vi "Filter Names by Suffix.vi"(8 "Error In":errorcluster, 9 "Ignore File Suffix Array":string[](array[string]), 11 "File Names":string[](array[string])) -> (0 "Error Out":errorcluster, 3 "Filtered File Names":string[](array[string]))   [LabVIEW 2021, in "Files.lvlib"]
uses:
  Files.lvlib
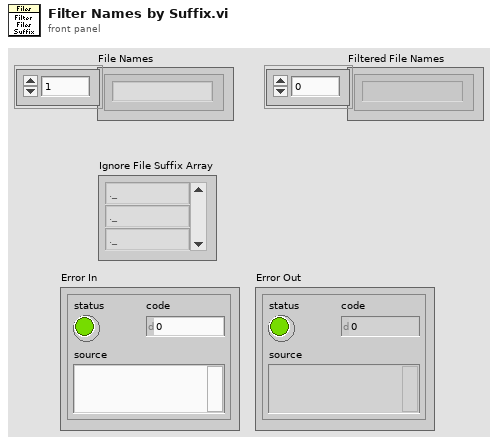
[diagram p1: front panel]
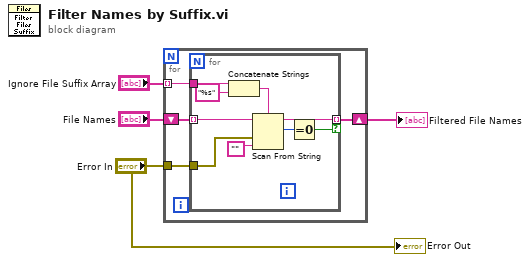
[diagram p0: block diagram]
diagram:
  n1 = for {
    shift-right: [w5] -> w2
    shift-left: "File Names" -> [w7]
    tunnel: "Ignore File Suffix Array" -> [w8] mode=indexing
    tunnel: "Error In" -> [w6]
    n2 = for {
      tunnel: w8 -> [w16]
      tunnel: w7 -> [w17] mode=indexing
      tunnel: w6 -> [w13]
      tunnel: [w10] -> w5 mode=indexing if=w9
      n3 = Concatenate Strings(w16, "%s" ("string")) -> (w14:string)
      n4 = Scan From String(format string=w14, input string=w17, error in=w13, default 1="") -> (remaining string=w10:string, offset past scan=w11:u32)  [unwired: 2 in, 1 out]
      n5 = Equal To 0?(x=w11) -> (x = 0?=w9:bool)
    }
  }
  "Filtered File Names" <- w2
  "Error Out" <- "Error In"
